vi "Formatted File Info.vi"(2 "Options":T1={"Name Bold"=TRUE, "Name Color"=0, "Include TimeStamp"=TRUE, "Time Format"="  %<%Y-%m-%d %H:%M>T", "TimeStamp Color"=10027008, "Include Size"=FALSE, "Size Format"="  %d", "Size Color"=255}, 3 "Path":path, 4 "Error In":errorcluster) -> (0 "Formatted String":string, 1 "Error Out":errorcluster)   [LabVIEW 2018]
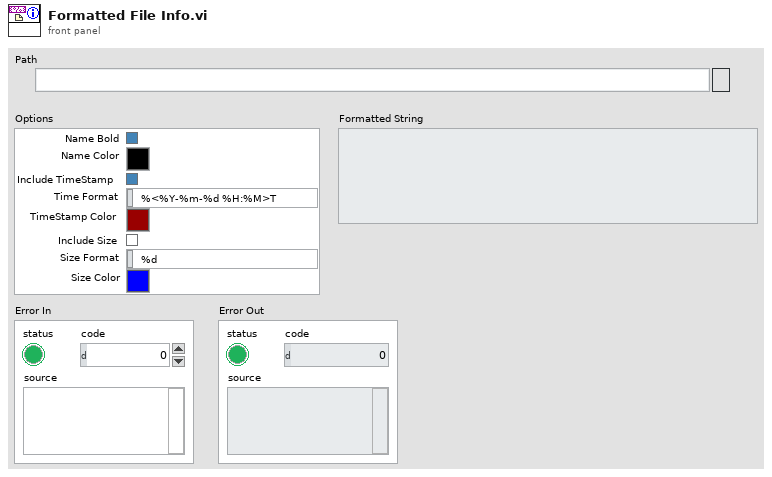
[diagram p1: front panel]
types:
  T1 = cluster{"Name Bold":bool, "Name Color":u32, "Include TimeStamp":bool, "Time Format":string, "TimeStamp Color":u32, "Include Size":bool, "Size Format":string, "Size Color":u32}
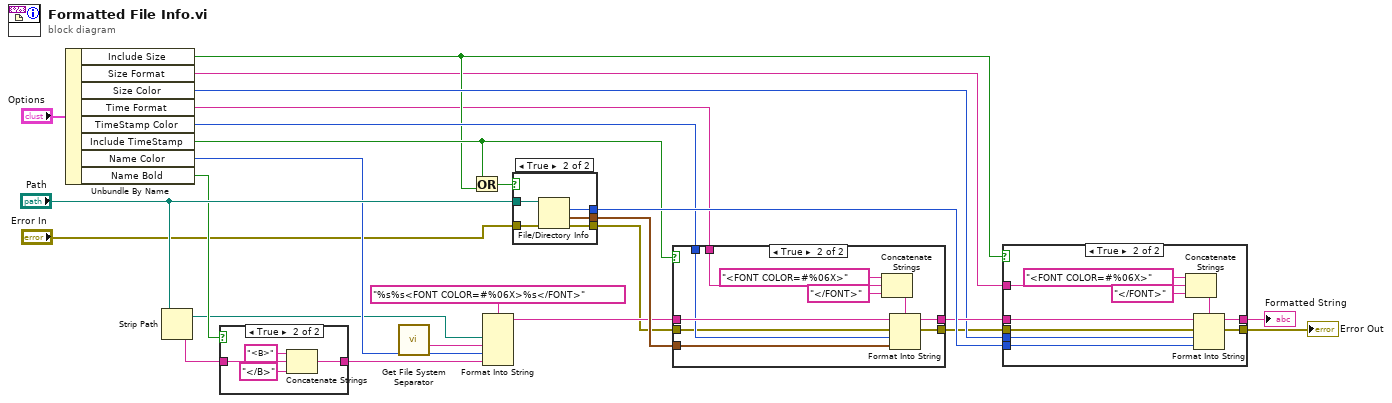
[diagram p0: block diagram]
diagram:
  n1 = Unbundle By Name("Options") -> ("Include Size"=w8:bool, "Size Format"=w4:string, "Size Color"=w10:u32, "Time Format"=w5:string, "TimeStamp Color"=w9:u32, "Include TimeStamp"=w14:bool, "Name Color"=w21:u32, "Name Bold"=w22:bool)
  n2 = Strip Path(path="Path") -> (stripped path=w15:path, name=w1:string)
  n3 = case shown="True" w22 {
    tunnel: w1 -> [w26 w30]
    tunnel: [w26 w27] -> w19
    frame False {
    }
    frame True {
      n4 = Concatenate Strings("<B>" ("string"), w30, "</B>" ("string")) -> (w27:string)
    }
  }
  n5 = call <vilib>:"Get File System Separator.vi"() -> ("Path Separator"=w16:string)
  n6 = Or(x=w14, y=w8) -> (x .or. y?=w23:bool)
  n7 = Format Into String(format string="%s%s<FONT COLOR=#%06X>%s</FONT>", w15, w16, w21, w19) -> (resulting string=w12:string)  [unwired: 2 in, 1 out]
  n8 = case shown="True" w23 {
    tunnel: [_ w36] -> w13
    tunnel: "Path" -> [_ w35]
    tunnel: [_ w34] -> w17
    tunnel: "Error In" -> [w31 w33]
    tunnel: [w31 w32] -> w6
    frame False {
    }
    frame True {
      n9 = File/Directory Info(path=w35, error in=w33) -> (size=w34:i64, last mod=w36:timestamp, error out=w32:errorcluster)  [unwired: 4 out]
    }
  }
  n10 = case shown="True" w14 {
    tunnel: w13 -> [_ w41]
    tunnel: w12 -> [w38 w48]
    tunnel: [w38 w46] -> w11
    tunnel: w5 -> [_ w42]
    tunnel: w9 -> [_ w45]
    tunnel: w6 -> [w37 w40]
    tunnel: [w37 w39] -> w3
    frame False {
    }
    frame True {
      n11 = Concatenate Strings("<FONT COLOR=#%06X>" ("format string"), w42, "</FONT>" ("string")) -> (w44:string)
      n12 = Format Into String(format string=w44, initial string=w48, error in=w40, w45, w41) -> (resulting string=w46:string, error out=w39:errorcluster)
    }
  }
  n13 = case shown="True" w8 {
    tunnel: w17 -> [_ w60]
    tunnel: w10 -> [_ w59]
    tunnel: w11 -> [w50 w58]
    tunnel: [w50 w57] -> w7
    tunnel: w4 -> [_ w53]
    tunnel: w3 -> [w49 w52]
    tunnel: [w49 w51] -> w2
    frame False {
    }
    frame True {
      n14 = Concatenate Strings("<FONT COLOR=#%06X>" ("format string"), w53, "</FONT>" ("string")) -> (w54:string)
      n15 = Format Into String(format string=w54, initial string=w58, error in=w52, w59, w60) -> (resulting string=w57:string, error out=w51:errorcluster)
    }
  }
  "Error Out" <- w2
  "Formatted String" <- w7
